vi "YJoystick_Dell.vi"(10 "Left X-Axis":dbl, 11 "Left Y-Axis":dbl) -> (2 "Left Motor":dbl, 3 "Right Motor":dbl)   [LabVIEW 2013]
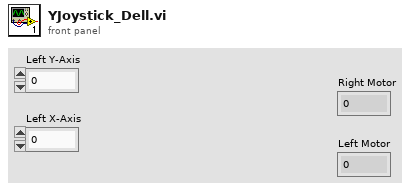
[diagram p1: front panel]
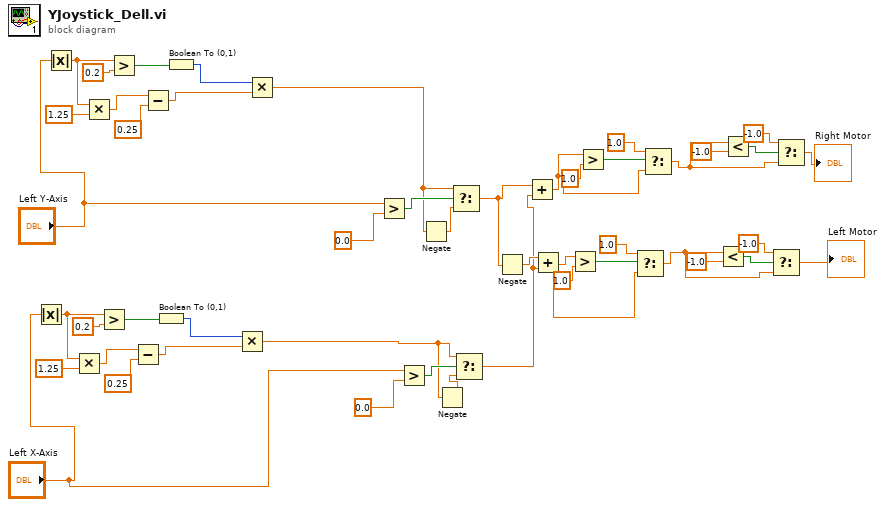
[diagram p0: block diagram]
diagram:
  n1 = Absolute Value(x="Left X-Axis") -> (abs(x)=w33:dbl)
  n2 = Absolute Value(x="Left Y-Axis") -> (abs(x)=w46:dbl)
  n3 = Multiply(x=w33, y=1.25) -> (x*y=w31:dbl)
  n4 = Multiply(x=w46, y=1.25) -> (x*y=w44:dbl)
  n5 = Greater?(x=w33, y=0.2) -> (0:w29:bool)
  n6 = Greater?(x=w46, y=0.2) -> (0:w42:bool)
  n7 = Subtract(x=w31, y=0.25) -> (x-y=w27:dbl)
  n8 = Subtract(x=w44, y=0.25) -> (x-y=w40:dbl)
  n9 = Boolean To (0,1)(Boolean=w29) -> (0, 1=w28:i16)
  n10 = Boolean To (0,1)(Boolean=w42) -> (0, 1=w41:i16)
  n11 = Multiply(x=w28, y=w27) -> (x*y=w14:dbl)
  n12 = Multiply(x=w41, y=w40) -> (x*y=w36:dbl)
  n13 = Greater?(x="Left Y-Axis", y=0.0) -> (0:w38:bool)
  n14 = Greater?(x="Left X-Axis", y=0.0) -> (0:w15:bool)
  n15 = Negate(x=w36) -> (-x=w35:dbl)
  n16 = Negate(x=w14) -> (-x=w13:dbl)
  n17 = Select(t=w36, s=w38, f=w35) -> (s? t:f=w26:dbl)
  n18 = Select(t=w14, s=w15, f=w13) -> (s? t:f=w12:dbl)
  n19 = Negate(x=w26) -> (-x=w25:dbl)
  n20 = Add(x=w26, y=w12) -> (x+y=w21:dbl)
  n21 = Add(x=w25, y=w12) -> (x+y=w17:dbl)
  n22 = Greater?(x=w17, y=1.0) -> (0:w19:bool)
  n23 = Greater?(x=w21, y=1.0) -> (0:w23:bool)
  n24 = Select(t=1.0, s=w19, f=w17) -> (s? t:f=w6:dbl)
  n25 = Select(t=1.0, s=w23, f=w21) -> (s? t:f=w2:dbl)
  n26 = Less?(x=w6, y=-1.0) -> (x < y?=w9:bool)
  n27 = Less?(x=w2, y=-1.0) -> (x < y?=w4:bool)
  n28 = Select(t=-1.0, s=w9, f=w6) -> (s? t:f=→"Left Motor":dbl)
  n29 = Select(t=-1.0, s=w4, f=w2) -> (s? t:f=→"Right Motor":dbl)
